vi "Hello world 2.vi"() -> ()   [LabVIEW 2016]
panel:
  in  "message":string="Hello World!!! v2"
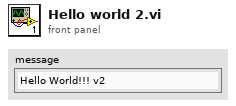
[diagram p1: front panel]
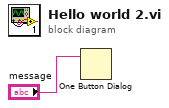
[diagram p0: block diagram]
diagram:
  n1 = One Button Dialog(message="message") -> ()  [unwired: 1 in, 1 out]
